vi "mod_Demodulate AM (SSB).vi"(0 "IQ data (complex)":cluster{"t0":dbl, "dt":dbl, "Y":cdb[]} {"Y" format="%.2f"; "dt" format="%.2f"; "t0" format="%.2f"}, 1 "costas loop parameters":T4={"Alpha"=0.001, "Beta"=0.0002}, 5 "modulation index":dbl=1.0 format="%.2f", 7 "pilot extraction filter":T3={"taps"=81, "approx freq. (Hz)"=0.0, "search (+/- % of Fsampl) "=0.25}, 11 "error in (no error)":errorcluster, 12 "suppress carrier ? (F)":bool, 13 "reset? (T)":bool=TRUE) -> (4 "AM demodulated waveform":waveform(dbl), 6 "Measurements":T2, 8 "filter information":T1 {"Pilot rejection filter"."df" format="%.2p"; "Pilot rejection filter"."f0" format="%.2p"; "Pilot rejection filter"."Mag H(w)" format="%.2p"; "Pilot extraction filter"."df" format="%.2p"; "Pilot extraction filter"."f0" format="%.2p"; "Pilot extraction filter"."Mag H(w)" format="%.2p"}, 15 "error out":errorcluster)   [LabVIEW 2020, in "niAMT.lvlib"]
uses:
  <vilib>/addons/Modulation/niAMT.lvlib
  <vilib>/addons/Modulation/Analog/controls/mod_Costas loop parameters.ctl
  <vilib>/addons/Modulation/Analog/controls/mod_AM pilot extraction filter.ctl
  <vilib>/addons/Modulation/Analog/controls/mod_AM Measurements.ctl
  <vilib>/addons/Modulation/Analog/controls/mod_AM pilot filter info.ctl
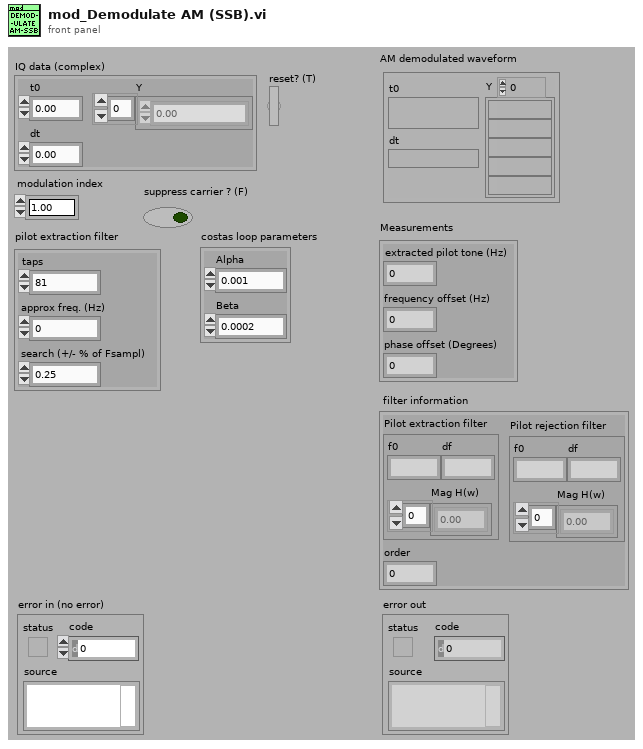
[diagram p1: front panel]
types:
  T1 = typedef "niAMT.lvlib/mod_AM pilot filter info.ctl" = cluster{"Pilot extraction filter":cluster{"f0":dbl, "df":dbl, "Mag H(w)":dbl[]}, "order":i32, "Pilot rejection filter":cluster{"f0":dbl, "df":dbl, "Mag H(w)":dbl[]}}
  T2 = typedef "niAMT.lvlib/mod_AM Measurements.ctl" = cluster{"extracted pilot tone (Hz)":dbl, "phase offset (Degrees)":dbl, "frequency offset (Hz)":dbl}
  T3 = typedef "niAMT.lvlib/mod_AM pilot extraction filter.ctl" = cluster{"taps":i32, "approx freq. (Hz)":dbl, "search (+/- % of Fsampl) ":dbl}
  T4 = typedef "niAMT.lvlib/mod_Costas loop parameters.ctl" = cluster{"Alpha":dbl, "Beta":dbl}
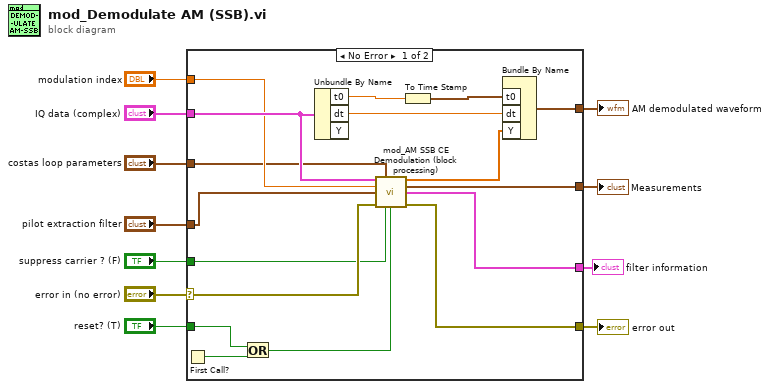
[diagram p0: block diagram]
diagram:
  n1 = case shown="No Error" "error in (no error)" {
    selector: "error in (no error)" -> [w25 w29]
    tunnel: [w24 w29] -> w10
    tunnel: "IQ data (complex)" -> [w19 _]
    tunnel: "modulation index" -> [w18 _]
    tunnel: "reset? (T)" -> [w23 _]
    tunnel: [w20 _] -> w6
    tunnel: "suppress carrier ? (F)" -> [w15 _]
    tunnel: "costas loop parameters" -> [w16 _]
    tunnel: "pilot extraction filter" -> [w14 _]
    tunnel: [w13 _] -> w2
    tunnel: [w12 _] -> w1
    frame No Error {
      n2 = First Call?() -> (First Call?: T/F=w22:bool)
      n3 = Or(x=w23, y=w22) -> (x .or. y?=w21:bool)
      n4 = Unbundle By Name(w19) -> ("t0"=w27:dbl, "dt"=w26:dbl)  [unwired: 1 out]
      n5 = call <vilib>:"mod_AM SSB CE Demodulation (block processing).vi"("input complex waveform"=w19, "costas loop parameters"=w16, "modulation index"=w18, "pilot extraction filter"=w14, "error in (no error)"=w25, "suppress carrier ? (F)"=w15, "reset? (T)"=w21) -> ("recovered message signal"=w17:dbl[], "measurements"=w13:T2, "filter information"=w12:T1, "error out"=w24:errorcluster)  [unwired: 3 in, 2 out]
      n6 = To Time Stamp(1:w27) -> (0:w28:timestamp)
      n7 = Bundle By Name("t0"=w28, "dt"=w26, "Y"=w17) -> (w20:waveform(dbl))  [unwired: 1 out]
    }
    frame Error {
    }
  }
  "error out" <- w10
  "AM demodulated waveform" <- w6
  "Measurements" <- w2
  "filter information" <- w1
